vi "Create_1.vi"(8 "error in (no error)":errorcluster, 11 "minimum log level (Info)":T1=enum."Info") -> (0 "error out":errorcluster)   [LabVIEW 2018]
uses:
  src/api/logger_class/Log Levels.ctl
  src/api/logger_class/Logger.lvclass
panel:
  # "Connector Pane"
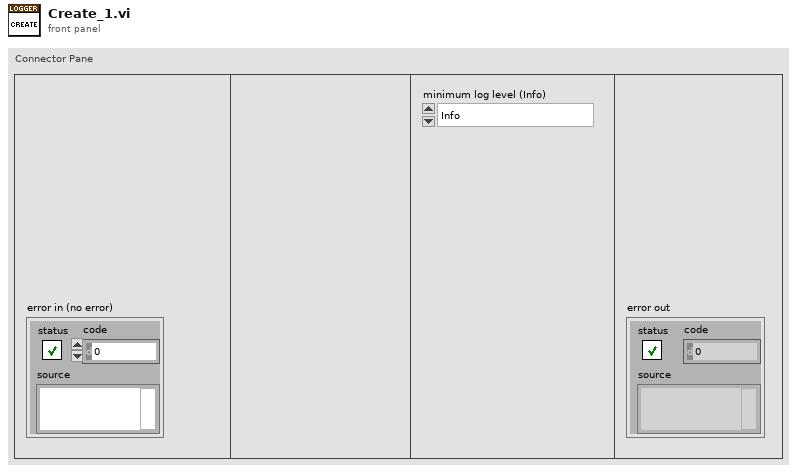
[diagram p1: front panel]
types:
  T1 = typedef "GLog.lvlib/Logger.lvclass/Log Levels.ctl" = enum16{"Trace", "Debug", "Info", "Warning", "Error", "Critical"}
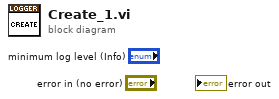
[diagram p0: block diagram]
diagram:
